vi "Digitizer_config_read.vi"(0 "Resource Name":string, 5 "Channel Name":string="0", 7 "Trigger settings":T2={"trigger level"=30.0, "trigger type"=enum."Edge", "Trigger Source"=enum."Channel 0", "Trigger Slope"=enum."Positive"} {"trigger level" format="%.2f"}, 9 "Vertical Settings":T3={"vertical coupling"=enum."DC", "probe attenuation"=20.0, "vertical range"=120.0, "vertical offset"=0.0} {"vertical offset" format="%.4f"; "vertical range" format="%.2f"; "probe attenuation" format="%.1f"}, 12 "Horizontal Settings":T1={"number of records"=1, "reference position"=50.0, "min record length"=50000, "min sample rate"=200000.0, "enforce realtime"=FALSE, "maximum input frequency"=0.0} {"maximum input frequency" format="%.2f"; "min sample rate" step=1000000.0 format="%.0p"; "reference position" format="%.1f"; "number of records" step=1}) -> (4 "Test Passed?":bool, 6 "Error message":string, 8 "Digitizer Error":bool, 10 "Plot":dbl[](array[numeric]), 15 "error out":errorcluster)   [LabVIEW 2010]
uses:
  <instrlib>/niScope/Acquire/niScope Multi Read Cluster.vi
  <instrlib>/niScope/Configure/Trigger/niScope Configure Trigger Edge.vi
  <instrlib>/niScope/Configure/Trigger/niScope Configure Trigger Digital.vi
  <instrlib>/niScope/Configure/Trigger/niScope Configure Trigger Immediate.vi
panel:
  out "actual sample rate":dbl=50000.0 caption="Actual Sample Rate" format="%.3p"
  out "actual record length":i32=50000 caption="Actual Record Length"
  out "Waveform Graph":T4(graph)=[{"relativeInitialX"=-0.5, "xIncrement"=2e-05, "wfm"=array[50000 elements]}]
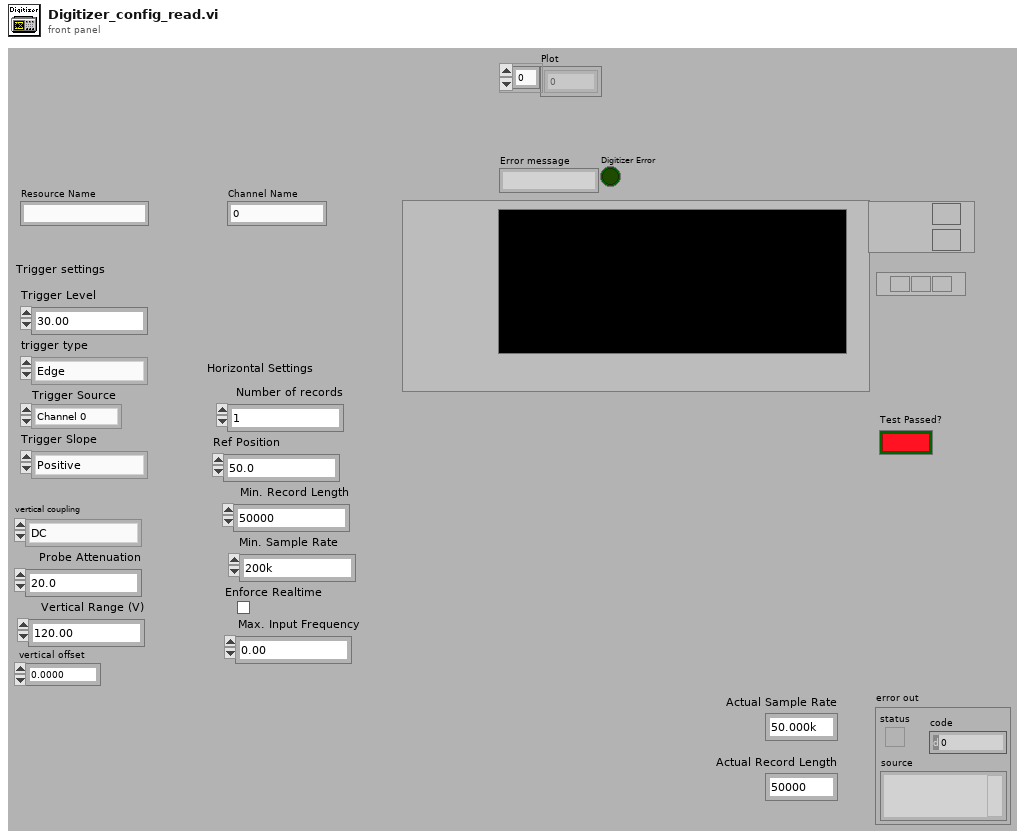
[diagram p1: front panel]
types:
  T1 = cluster{"number of records":i32, "reference position":dbl, "min record length":i32, "min sample rate":dbl, "enforce realtime":bool, "maximum input frequency":dbl}
  T2 = cluster{"trigger level":dbl, "trigger type":enum16{"Edge", "Digital", "Immediate"}, "Trigger Source":enum8{"Immediate", "Channel 0", "Channel 1", "Channel 2", "Channel 3", "Channel 4", "Channel 5", "Channel 6", "Channel 7", "External TRIG", "Software Trigger", "RTSI 0", "RTSI 1", "RTSI 2", "RTSI 3", "RTSI 4", "RTSI 5", "RTSI 6", "PFI 0", "PFI 1", "PFI 2", "PXI Star Trigger"}, "Trigger Slope":enum16{"Positive", "Negative"}}
  T3 = cluster{"vertical coupling":enum16{"AC", "DC", "Ground"}, "probe attenuation":dbl, "vertical range":dbl, "vertical offset":dbl}
  T4 = cluster{"relativeInitialX":dbl, "xIncrement":dbl, "wfm":dbl[]}[]
  T5 = enum8{"Immediate", "Channel 0", "Channel 1", "Channel 2", "Channel 3", "Channel 4", "Channel 5", "Channel 6", "Channel 7", "External TRIG", "Software Trigger", "RTSI 0", "RTSI 1", "RTSI 2", "RTSI 3", "RTSI 4", "RTSI 5", "RTSI 6", "PFI 0", "PFI 1", "PFI 2", "PXI Star Trigger"}
  T6 = cluster{"relativeInitialX":dbl, "xIncrement":dbl, "wfm":dbl[]}
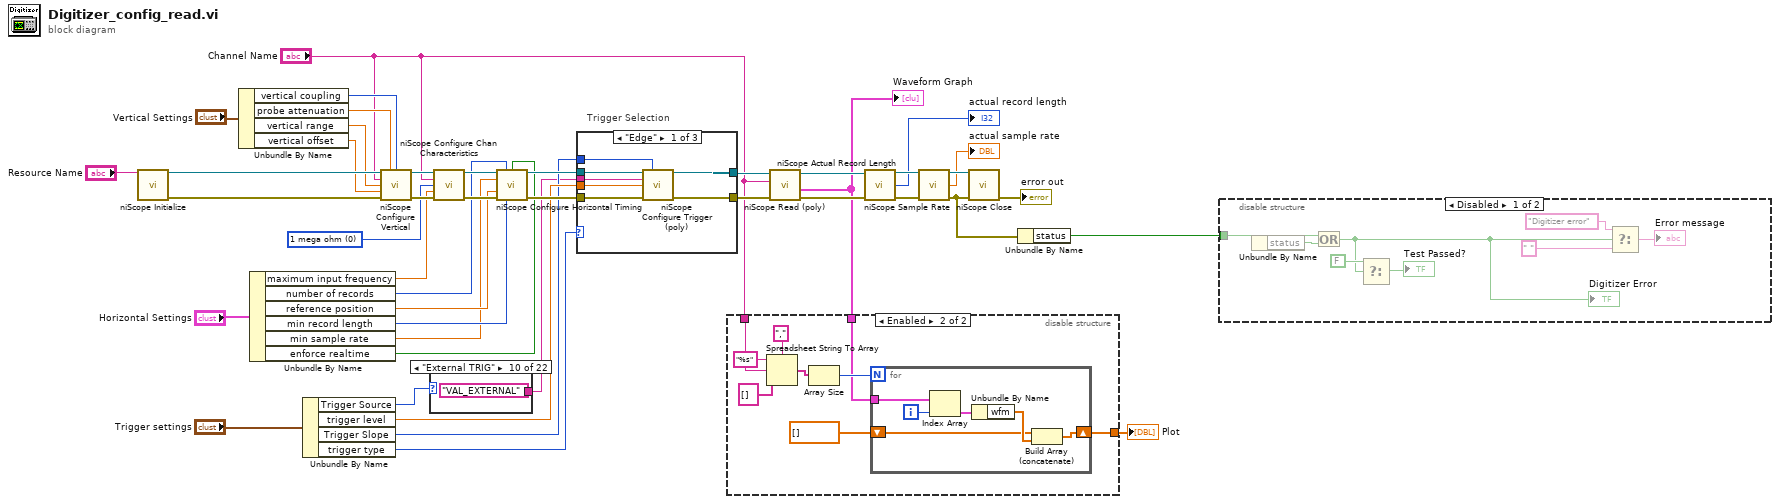
[diagram p0: block diagram]
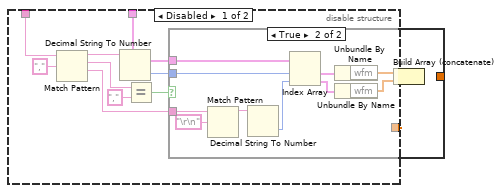
[diagram p2: hidden frame]
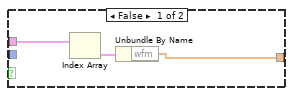
[diagram p3: hidden frame]
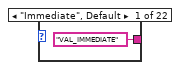
[diagram p5: hidden frame]
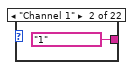
[diagram p6: hidden frame]
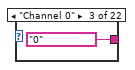
[diagram p7: hidden frame]
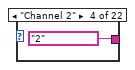
[diagram p8: hidden frame]
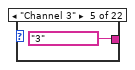
[diagram p9: hidden frame]
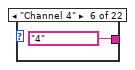
[diagram p10: hidden frame]
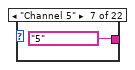
[diagram p11: hidden frame]
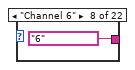
[diagram p12: hidden frame]
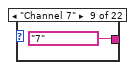
[diagram p13: hidden frame]
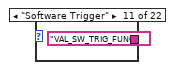
[diagram p14: hidden frame]
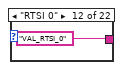
[diagram p15: hidden frame]
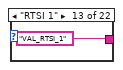
[diagram p16: hidden frame]
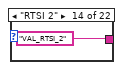
[diagram p17: hidden frame]
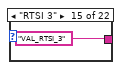
[diagram p18: hidden frame]
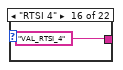
[diagram p19: hidden frame]
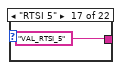
[diagram p20: hidden frame]
diagram:
  w29 = u32 0 items=["1 mega ohm", "75 ohms", "50 ohms"] ("input impedance")
  n1 = call <instrlib>:"niScope Initialize.vi"("resource name"="Resource Name") -> ("instrument handle"=w42:refnum<k15>, "error out"=w1:errorcluster)  [unwired: 13 in]
  n2 = Unbundle By Name("Vertical Settings") -> ("vertical coupling"=w22:enum16{"AC", "DC", "Ground"}, "probe attenuation"=w21:dbl, "vertical range"=w20:dbl, "vertical offset"=w8:dbl)
  n3 = Unbundle By Name("Horizontal Settings") -> ("maximum input frequency"=w9:dbl, "number of records"=w14:i32, "reference position"=w13:dbl, "min record length"=w12:i32, "min sample rate"=w11:dbl, "enforce realtime"=w10:bool)
  n4 = Unbundle By Name("Trigger settings") -> ("Trigger Source"=w7:T5, "trigger level"=w18:dbl, "Trigger Slope"=w17:enum16{"Positive", "Negative"}, "trigger type"=w16:enum16{"Edge", "Digital", "Immediate"})
  n5 = call <instrlib>:"niScope Configure Vertical.vi"("instrument handle"=w42, "probe attenuation"=w21, "vertical coupling"=w22, "channels"="Channel Name", "vertical range"=w20, "vertical offset"=w8, "error in"=w1) -> ("instrument handle out"=w33:refnum<k15>, "error out"=w32:errorcluster)  [unwired: 7 in]
  n6 = case shown="\"External TRIG\"" w7 {
    tunnel: ["VAL_IMMEDIATE" ("trigger source") "1" ("trigger source") "0" ("trigger source") "2" ("trigger source") "3" ("trigger source") "4" ("trigger source") "5" ("trigger source") "6" ("trigger source") "7" ("trigger source") "VAL_EXTERNAL" ("trigger source") "VAL_SW_TRIG_FUNC" ("trigger source") "VAL_RTSI_0" ("trigger source") "VAL_RTSI_1" ("trigger source") "VAL_RTSI_2" ("trigger source") "VAL_RTSI_3" ("trigger source") "VAL_RTSI_4" ("trigger source") "VAL_RTSI_5" ("trigger source") "VAL_RTSI_6" ("trigger source") "VAL_PFI_0" ("trigger source") "VAL_PFI_1" ("trigger source") "VAL_PFI_2" ("trigger source") "VAL_PXI_STAR" ("trigger source")] -> w6
    frame "Immediate", Default {
    }
    frame "Channel 1" {
    }
    frame "Channel 0" {
    }
    frame "Channel 2" {
    }
    frame "Channel 3" {
    }
    frame "Channel 4" {
    }
    frame "Channel 5" {
    }
    frame "Channel 6" {
    }
    frame "Channel 7" {
    }
    frame "External TRIG" {
    }
    frame "Software Trigger" {
    }
    frame "RTSI 0" {
    }
    frame "RTSI 1" {
    }
    frame "RTSI 2" {
    }
    frame "RTSI 3" {
    }
    frame "RTSI 4" {
    }
    frame "RTSI 5" {
    }
    frame "RTSI 6" {
    }
    frame "PFI 0" {
    }
    frame "PFI 1" {
    }
    frame "PFI 2" {
    }
    frame "PXI Star Trigger" {
    }
  }
  n7 = call <instrlib>:"niScope Configure Chan Characteristics.vi"("instrument handle"=w33, "channels"="Channel Name", "input impedance"=w29, "maximum input frequency"=w9, "error in"=w32) -> ("instrument handle out"=w30:refnum<k15>, "error out"=w31:errorcluster)  [unwired: 9 in]
  n8 = call <instrlib>:"niScope Configure Horizontal Timing.vi"("instrument handle"=w30, "number of records"=w14, "enforce realtime"=w10, "min sample rate"=w11, "reference position"=w13, "error in"=w31, "min record length"=w12) -> ("instrument handle out"=w27:refnum<k15>, "error out"=w28:errorcluster)  [unwired: 7 in]
  n9 = case "Trigger Selection" shown="\"Edge\"" w16 {
    tunnel: w28 -> [w72 w78 w82]
    tunnel: [w68 w74 w79] -> w25
    tunnel: w27 -> [w71 w77 w81]
    tunnel: [w69 w75 w80] -> w26
    tunnel: w6 -> [w70 w76 _]
    tunnel: w18 -> [w67 _ _]
    tunnel: w17 -> [w66 w73 _]
    frame "Edge" {
      n10 = call-poly <instrlib>:"niScope Configure Trigger (poly).vi"("instrument handle"=w71, "trigger slope"=w66, "trigger source"=w70, "trigger level"=w67, "error in"=w72) -> ("instrument handle out"=w69:refnum<k15>, "error out"=w68:errorcluster)  [unwired: 9 in]
    }
    frame "Digital" {
      n11 = call-poly <instrlib>:"niScope Configure Trigger (poly).vi"("instrument handle"=w77, "trigger slope"=w73, "trigger source"=w76, "error in"=w78) -> ("instrument handle out"=w75:refnum<k15>, "error out"=w74:errorcluster)  [unwired: 10 in]
    }
    frame "Immediate", Default {
      n12 = call-poly <instrlib>:"niScope Configure Trigger (poly).vi"("instrument handle"=w81, "error in"=w82) -> ("instrument handle out"=w80:refnum<k15>, "error out"=w79:errorcluster)  [unwired: 12 in]
    }
  }
  n13 = call-poly <instrlib>:"niScope Read (poly).vi"("error in"=w25, "channels"="Channel Name", "instrument handle"=w26) -> ("error out"=w38:errorcluster, "waveform"=w2:T4, "instrument handle out"=w24:refnum<k15>)  [unwired: 5 in, 1 out]
  "Waveform Graph" <- w2
  n14 = disable-structure shown="Enabled" {
    disable-tunnel: "Channel Name" -> [w92 w112]
    disable-tunnel: [w84 w110] -> w3
    disable-tunnel: w2 -> [w83 w111]
    frame Disabled {
      n15 = Match Pattern(string=w92, regular expression=",") -> (before substring=w90:string, match substring=w89:string, after substring=w86:string)  [unwired: 1 in, 1 out]
      n16 = Decimal String To Number(string=w90) -> (number=w85:i32)  [unwired: 2 in, 1 out]
      n17 = Equal?(x=w89, y=",") -> (x = y?=w87:bool)
      n18 = case shown="True" w87 {
        tunnel: w86 -> [_ w105]
        tunnel: w83 -> [w94 w103]
        tunnel: [w93 w96] -> w84
        tunnel: w85 -> [_ w102]
        frame False {
          n19 = Index Array(array=w94) -> (element=w95:T6)  [unwired: 1 in]
          n20 = Unbundle By Name(w95) -> ("wfm"=w93:dbl[])
        }
        frame True {
          n21 = Match Pattern(string=w105, regular expression="\r\n") -> (before substring=w101:string)  [unwired: 1 in, 3 out]
          n22 = Decimal String To Number(string=w101) -> (number=w100:i32)  [unwired: 2 in, 1 out]
          n23 = Index Array(array=w103, index #1=w102, index #2=w100) -> (element #1=w104:T6, element #2=w99:T6)
          n24 = Unbundle By Name(w104) -> ("wfm"=w98:dbl[])
          n25 = Unbundle By Name(w99) -> ("wfm"=w97:dbl[])
          n26 = Build Array (concatenate)(w98, w97) -> (w96:dbl[])
        }
      }
    }
    frame Enabled {
      n27 = Spreadsheet String To Array(delimiter (Tab)=",", format string="%s", spreadsheet string=w112, array type (2D Dbl)=string[] []) -> (array=w113:string[])
      n28 = Array Size(array=w113) -> (size(s)=w114:i32)
      n29 = for {
        N: w114 -> [_]
        shift-right: [w118] -> w110
        shift-left: dbl[] [] -> [w117]
        tunnel: w111 -> [w116]
        i -> [w121]
        n30 = Index Array(array=w116, index=w121) -> (element=w120:T6)
        n31 = Unbundle By Name(w120) -> ("wfm"=w119:dbl[])
        n32 = Build Array (concatenate)(w117, w119) -> (w118:dbl[])
      }
    }
  }
  "Plot" <- w3
  n33 = call <instrlib>:"niScope Actual Record Length.vi"("instrument handle"=w24, "error in"=w38) -> ("instrument handle out"=w36:refnum<k15>, "actual record length"=→"actual record length":i32, "error out"=w35:errorcluster)  [unwired: 11 in]
  n34 = call <instrlib>:"niScope Sample Rate.vi"("instrument handle"=w36, "error in"=w35) -> ("instrument handle out"=w43:refnum<k15>, "actual sample rate"=→"actual sample rate":dbl, "error out"=w41:errorcluster)  [unwired: 11 in]
  n35 = call <instrlib>:"niScope Close.vi"("instrument handle"=w43, "error in"=w41) -> ("error out"=→"error out":errorcluster)  [unwired: 13 in]
  n36 = Unbundle By Name(w41) -> ("status"=w5:bool)
  n37 = disable-structure shown="Disabled" {
    disable-tunnel: w5 -> [w124 _]
    frame Disabled {
      n38 = Unbundle By Name() -> ("status"=w123:bool)  [unwired: 1 in]
      n39 = Or(x=w124, y=w123) -> (x .or. y?=w122:bool)
      "Digitizer Error" <- w122
      n40 = Select(t=FALSE, s=w122) -> (s? t:f=→"Test Passed?":bool)  [unwired: 1 in]
      n41 = Select(t="Digitizer error", s=w122, f=" ") -> (s? t:f=→"Error message":string)
    }
    frame Enabled {
    }
  }
